vi "test_pv.vi"() -> ()   [LabVIEW 2023]
uses:
  <vilib>/picture/picture.llb/Draw True-Color Pixmap.vi
  hl2ss_ulm.dll
panel:
  out "Pose":sgl[][](array[numeric])
  out "Video":picture
  out "packet":u64[](array[numeric])
  in  "stop":bool
  in  "Framerate":u8=30
  in  "Height":u16=360
  in  "Width":u16=640
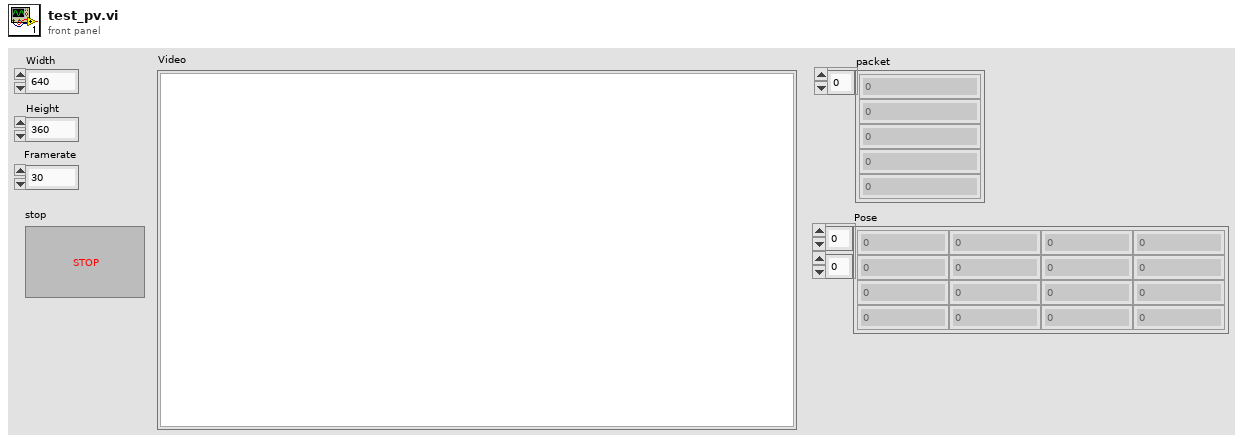
[diagram p1: front panel]
types:
  T1 = cluster{"enable_mrc":u8, "hologram_composition":u8, "recording_indicator":u8, "video_stabilization":u8, "blank_protected":u8, "show_mesh":u8, "shared":u8, "_reserved_0":u8, "global_opacity":sgl, "output_width":sgl, "output_height":sgl, "video_stabilization_length":u32, "hologram_perspective":u32, "_reserved_1":u32}
  T2 = cluster{"chunk":u64, "mode":u8, "_reserved_0":u8, "width":u16, "height":u16, "framerate":u8, "_reserved_1":u8, "divisor":u8, "profile":u8, "level":u8, "decoded format":u8, "bitrate":u32, "options_size":i64, "options_data":u64}
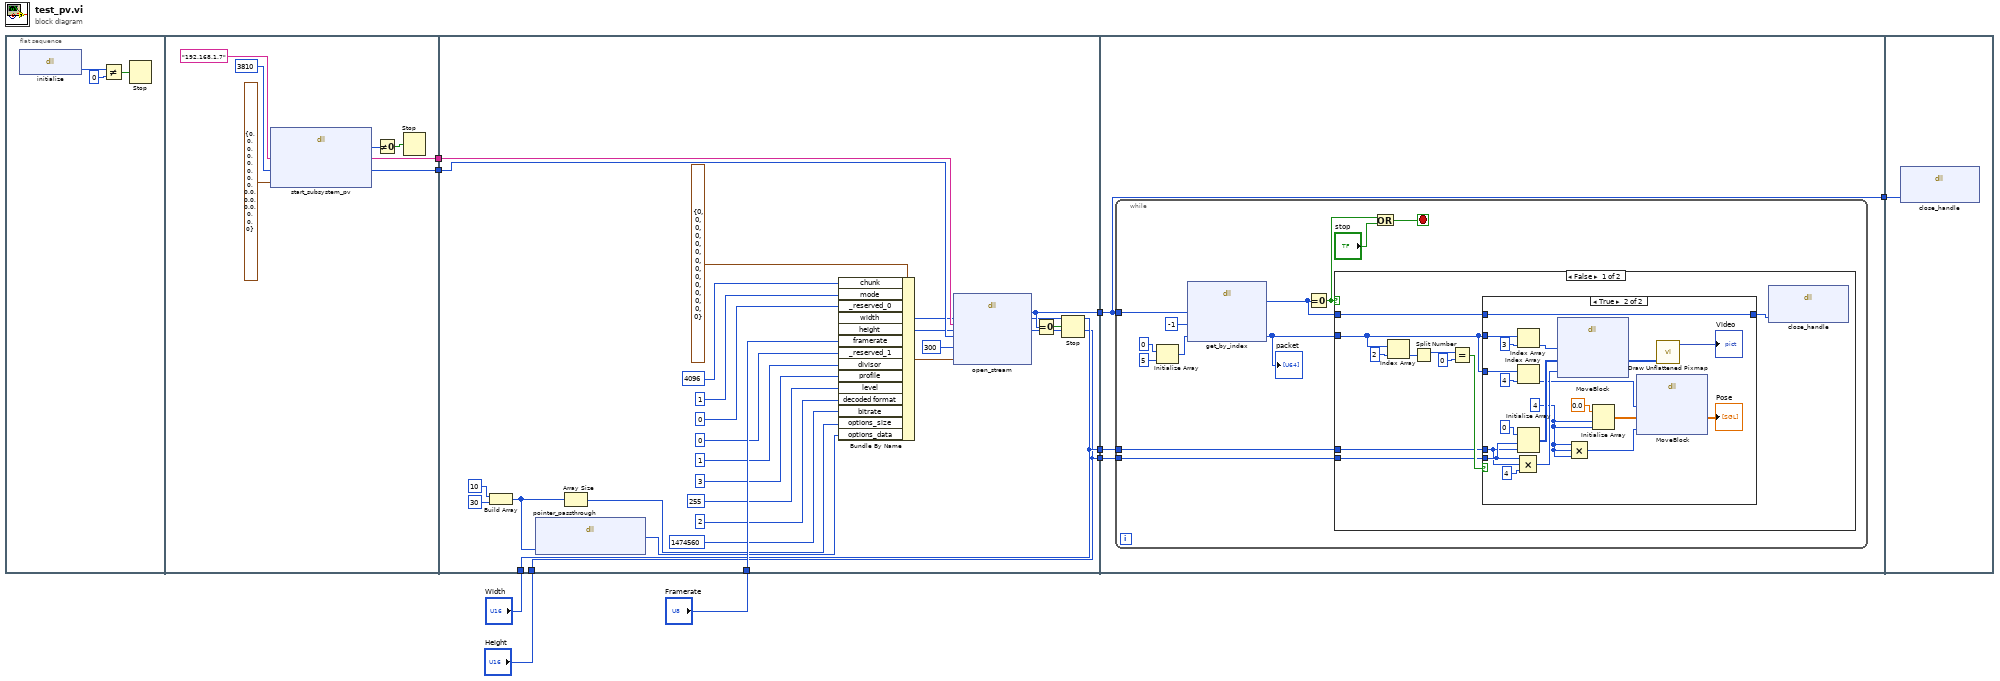
[diagram p0: block diagram]
diagram:
  n1 = flat-sequence {
    tunnel: [w17] -> w6
    tunnel: [w16] -> w5
    tunnel: "Width" -> [w21]
    tunnel: "Height" -> [w20]
    tunnel: "Framerate" -> [w33]
    tunnel: w6 -> [w43]
    tunnel: w5 -> [w42]
    tunnel: [w40] -> w4
    tunnel: [w21] -> w2
    tunnel: [w20] -> w1
    tunnel: w4 -> [w46]
    tunnel: [w46] -> w3
    tunnel: w2 -> [w45]
    tunnel: w1 -> [w44]
    tunnel: w3 -> [w90]
    frame #0 {
      n2 = dll-call lib="C:/Users/jcds/Documents/GitHub/hl2ss/extensions/client_labview/hl2ss_ulm.dll" fn="initialize"() -> ("return type"=w12:i32)  [unwired: 3 in, 2 out]
      n3 = Not Equal?(x=w12, y=0) -> (x != y?=w10:bool)
      n4 = Stop(stop? (T)=w10) -> ()
    }
    frame #1 {
      n5 = dll-call lib="C:/Users/jcds/Documents/GitHub/hl2ss/extensions/client_labview/hl2ss_ulm.dll" fn="start_subsystem_pv"("host"="192.168.1.7", "port"=u16 3810, "configuration"=T1 {"enable_mrc"=0, "hologram_composition"=0, "recording_indicator"=0, "video_stabilization"=0, "blank_protected"=0, "show_mesh"=0, "shared"=0, "_reserved_0"=0, "global_opacity"=0.0, "output_width"=0.0, "output_height"=0.0, "video_stabilization_length"=0, "hologram_perspective"=0, "_reserved_1"=0} ("Cluster")) -> ("return type"=w14:i32, "host"=w17:string, "port"=w16:u16)  [unwired: 4 in, 2 out]
      n6 = Not Equal To 0?(x=w14) -> (x != 0?=w15:bool)
      n7 = Stop(stop? (T)=w15) -> ()
    }
    frame #2 {
      n8 = Build Array(u64 10, u64 30) -> (w22:u64[])
      n9 = dll-call lib="C:/Users/jcds/Documents/GitHub/hl2ss/extensions/client_labview/hl2ss_ulm.dll" fn="pointer_passthrough"("p"=w22) -> ("return type"=w25:u64)  [unwired: 4 in, 2 out]
      n10 = Array Size(array=w22) -> (size(s)=w26:i32)
      n11 = Bundle By Name(cluster=T2 {"chunk"=0, "mode"=0, "_reserved_0"=0, "width"=0, "height"=0, "framerate"=0, "_reserved_1"=0, "divisor"=0, "profile"=0, "level"=0, "decoded format"=0, "bitrate"=0, "options_size"=0, "options_data"=0} ("Cluster"), "chunk"=u64 4096, "mode"=u8 1, "_reserved_0"=u8 0, "width"=w21, "height"=w20, "framerate"=w33, "_reserved_1"=u8 0, "divisor"=u8 1, "profile"=u8 3, "level"=u8 255, "decoded format"=u8 2, "bitrate"=u32 1474560, "options_size"=w26, "options_data"=w25) -> (w37:T2)
      n12 = dll-call lib="C:/Users/jcds/Documents/GitHub/hl2ss/extensions/client_labview/hl2ss_ulm.dll" fn="open_stream"("host"=w43, "port"=w42, "buffer_size"=u64 300, "configuration"=w37) -> ("return type"=w40:u64)  [unwired: 7 in, 2 out]
      n13 = Equal To 0?(x=w40) -> (x = 0?=w39:bool)
      n14 = Stop(stop? (T)=w39) -> ()
    }
    frame #3 {
      n15 = while {
        tunnel: w46 -> [w58]
        tunnel: w45 -> [w48]
        tunnel: w44 -> [w47]
        stop <- w52 stop-if-true
        n16 = Initialize Array(u64 0, 5 ("dimension size")) -> (w54:u64[])
        n17 = dll-call lib="C:/Users/jcds/Documents/GitHub/hl2ss/extensions/client_labview/hl2ss_ulm.dll" fn="get_by_index"("handle"=w58, "frame_stamp"=i64 -1, "packet"=w54) -> ("return type"=w50:u64, "packet"=w49:u64[])  [unwired: 5 in, 2 out]
        "packet" <- w49
        n18 = Equal To 0?(x=w50) -> (x = 0?=w51:bool)
        n19 = case shown="False" w51 {
          tunnel: w50 -> [w62 _]
          tunnel: w49 -> [w61 _]
          tunnel: w48 -> [w60 _]
          tunnel: w47 -> [w59 _]
          frame False {
            n20 = Index Array(array=w61, index=2) -> (element=w67:u64)
            n21 = Split Number(x=w67) -> (hi(x)=w66:u32)  [unwired: 1 out]
            n22 = Equal?(x=w66, y=u32 0) -> (x = y?=w64:bool)
            n23 = case shown="True" w64 {
              tunnel: [w69 w89] -> w63
              tunnel: w62 -> [w69 w89]
              tunnel: w61 -> [_ w88]
              tunnel: w61 -> [_ w86]
              tunnel: w60 -> [_ w77]
              tunnel: w59 -> [_ w78]
              frame False {
              }
              frame True {
                w72 = 4 ("dimension size")
                n24 = Index Array(array=w88, index=3) -> (element=w83:u64)
                n25 = Index Array(array=w86, index=4) -> (element=w75:u64)
                n26 = Initialize Array(u32 0, w78, w77) -> (w80:u32[][])
                n27 = Compound Arithmetic op=MULTIPLY(w78, w77, u32 4 ("value")) -> (w82:u32)
                n28 = dll-call lib="LabVIEW" fn="MoveBlock"("ps"=w83, "pd"=w80, "size"=w82) -> ("pd"=w76:u32[][])  [unwired: 6 in, 2 out]
                n29 = Compound Arithmetic op=MULTIPLY(w72, w72, w72) -> (w71:i32)
                n30 = Initialize Array(sgl 0.0 ("element"), w72, w72) -> (w73:sgl[][])
                n31 = dll-call lib="LabVIEW" fn="MoveBlock"("ps"=w75, "pd"=w73, "size"=w71) -> ("pd"=→"Pose":sgl[][])  [unwired: 6 in, 2 out]
                n32 = call-poly <vilib>:"Draw Unflattened Pixmap.vi"("data (RGB format)"=w76) -> ("new picture"=→"Video":picture)  [unwired: 8 in]
              }
            }
            n33 = dll-call lib="C:/Users/jcds/Documents/GitHub/hl2ss/extensions/client_labview/hl2ss_ulm.dll" fn="close_handle"("handle"=w63) -> ()  [unwired: 5 in, 2 out]
          }
          frame True {
          }
        }
        n34 = Or(x=w51, y="stop") -> (x .or. y?=w52:bool)
      }
    }
    frame #4 {
      n35 = dll-call lib="C:/Users/jcds/Documents/GitHub/hl2ss/extensions/client_labview/hl2ss_ulm.dll" fn="close_handle"("handle"=w90) -> ()  [unwired: 5 in, 2 out]
    }
  }
